vi "Pre Launch Init.vi"(11 "Controller in":refnum<class "Controller.lvclass">) -> (0 "error out":errorcluster, 3 "Controller out":refnum<class "Controller.lvclass">)   [LabVIEW 2022 SP3, in "Controller.lvlib" / "Controller.lvclass"]
doc: "(<B>Filename</B>: Actor Framework.lvlib:Actor.lvclass:Pre Launch Init.vi)\n\nDefines behavior that occurs after the Launch Nested Actor method is invoked but before the actor's Actor Core method begins running.\n\nBy default, this method does nothing. A descendant class may override it to define behavior."
uses:
  Controller.lvclass
  Controller.lvclass/Controller.ctl
  <vilib>/ActorFramework/Actor/Actor.lvclass
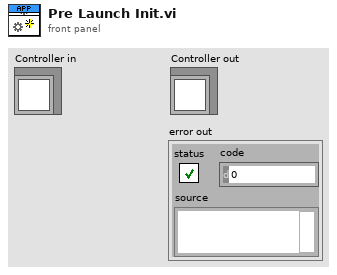
[diagram p1: front panel]
types:
  T1 = cluster{"Config File ":path, "Configuration":path, "Event Log":path, "Error Log":path}
  T2 = enum16{"open", "replace", "create", "open or create", "replace or create", "replace or create with confirmation"}
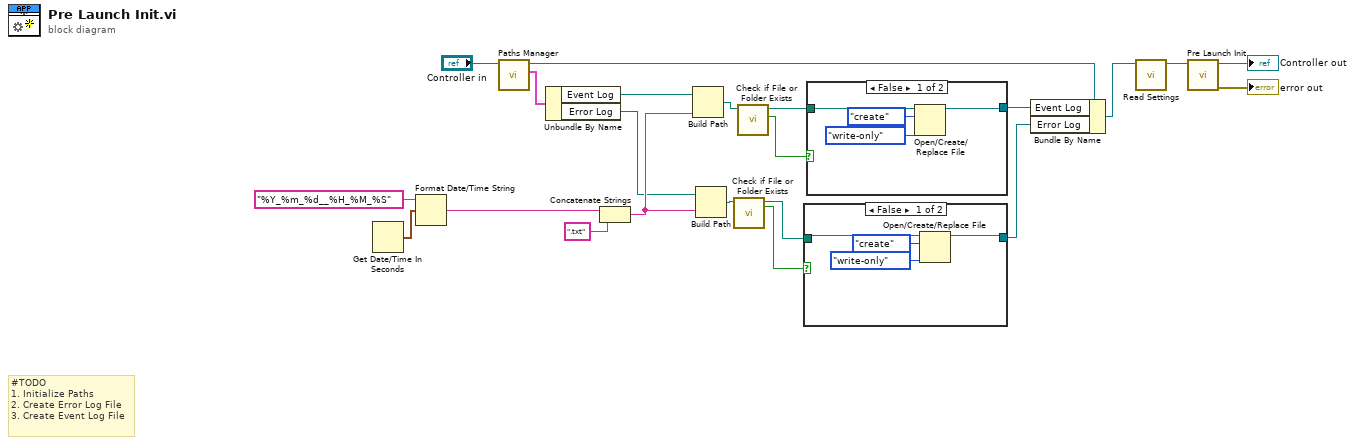
[diagram p0: block diagram]
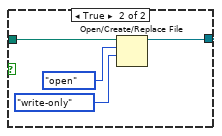
[diagram p2: hidden frame]
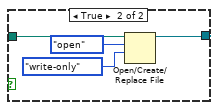
[diagram p3: hidden frame]
diagram:
  # "#TODO \n1. Initialize Paths\n2. Create Error Log File\n3. Create Event Log File"
  n1 = Get Date/Time In Seconds() -> (seconds since 1Jan1904=w2:timestamp)
  n2 = Format Date/Time String(time format string (%c)="%Y_%m_%d__%H_%M_%S", seconds (now)=w2) -> (date/time string=w1:string)  [unwired: 1 in]
  n3 = call "Paths Manager.vi"("Controller in"="Controller in") -> ("Paths"=w17:T1, "Controller out"=w18:refnum<class "Controller.lvclass">)  [unwired: 8 in, 1 out]
  n4 = Unbundle By Name(w17) -> ("Event Log"=w5:path, "Error Log"=w4:path)
  n5 = Concatenate Strings(w1, ".txt" ("string")) -> (w7:string)
  n6 = Build Path(base path=w5, name or relative path=w7) -> (appended path=w16:path)
  n7 = Build Path(base path=w4, name or relative path=w7) -> (appended path=w13:path)
  n8 = call <vilib>:"Check if File or Folder Exists.vi"("path"=w13) -> ("file or folder exists?"=w11:bool, "dup path"=w12:path)  [unwired: 8 in, 1 out]
  n9 = call <vilib>:"Check if File or Folder Exists.vi"("path"=w16) -> ("file or folder exists?"=w15:bool, "dup path"=w14:path)  [unwired: 8 in, 1 out]
  n10 = case shown="False" w11 {
    tunnel: [w26 w30] -> w10
    tunnel: w12 -> [w25 w27]
    frame False {
      n11 = Open/Create/Replace File(file path (use dialog)=w25, operation (0:open)=T2."create", access (0:read/write)=enum16{"read/write", "read-only", "write-only"}."write-only") -> (refnum out=w26:refnum<file>)  [unwired: 3 in, 2 out]
    }
    frame True {
      n12 = Open/Create/Replace File(file path (use dialog)=w27, operation (0:open)=T2."open", access (0:read/write)=enum16{"read/write", "read-only", "write-only"}."write-only") -> (refnum out=w30:refnum<file>)  [unwired: 3 in, 2 out]
    }
  }
  n13 = case shown="False" w15 {
    tunnel: [w31 w38] -> w20
    tunnel: w14 -> [w34 w35]
    frame False {
      n14 = Open/Create/Replace File(file path (use dialog)=w34, operation (0:open)=T2."create", access (0:read/write)=enum16{"read/write", "read-only", "write-only"}."write-only") -> (refnum out=w31:refnum<file>)  [unwired: 3 in, 2 out]
    }
    frame True {
      n15 = Open/Create/Replace File(file path (use dialog)=w35, operation (0:open)=T2."open", access (0:read/write)=enum16{"read/write", "read-only", "write-only"}."write-only") -> (refnum out=w38:refnum<file>)  [unwired: 3 in, 2 out]
    }
  }
  n16 = Bundle By Name(cluster=w18, "Event Log"=w20, "Error Log"=w10) -> (w9:refnum<class "Controller.lvclass">)
  n17 = call "Read Settings.vi"("Controller in"=w9) -> ("Controller out"=w8:refnum<class "Controller.lvclass">)  [unwired: 8 in, 2 out]
  n18 = call-parent "Pre Launch Init.vi"("Actor in"=w8) -> ("error out"=→"error out":errorcluster, "Actor out"=→"Controller out":refnum<class "Controller.lvclass">)  [unwired: 9 in]
